vi "Get State Analyzer.vi"(8 "error in (no error)":errorcluster, 11 "Debugger in":refnum<class "Debugger.lvclass">) -> (0 "error out":errorcluster, 2 "Log":refnum<class "Debug State Analyzer.lvclass">, 3 "Debugger out":refnum<class "Debugger.lvclass">)   [LabVIEW 2020, in "Debugger.lvclass"]
uses:
  Debugger.lvclass
  State Analyzer/Debug State Analyzer.lvclass
  Debugger.lvclass/Debugger.ctl
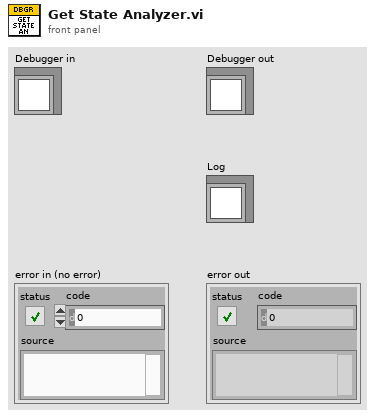
[diagram p1: front panel]
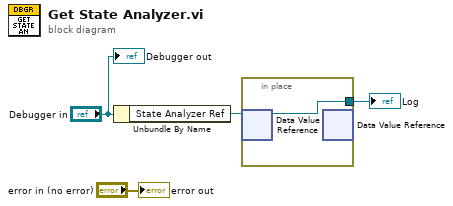
[diagram p0: block diagram]
diagram:
  n1 = Unbundle By Name("Debugger in") -> ("State Analyzer Ref"=w2:refnum<data-value>)
  n2 = in-place {
    in-place-border: [w5] -> w1
    n3 = in-place-dvr #1(w2) -> (w5:refnum<class "Debug State Analyzer.lvclass">)  [unwired: 1 out]
    n4 = in-place-dvr #1() -> ()  [unwired: 1 in, 2 out]
  }
  "Log" <- w1
  "Debugger out" <- "Debugger in"
  "error out" <- "error in (no error)"
